vi "niRFUtil FWK Check Floating Point Range.vi"(0 "Upper Limit":dbl format="%#_6p", 1 "Upper Limit epsilon":dbl=1e-08, 2 "Lower Limit epsilon":dbl=1e-08, 5 "Lower Limit":dbl format="%#_6p", 7 "Value":dbl format="%#_6p", 11 "error in (no error)":errorcluster) -> (4 "In Range?":bool, 15 "error out":errorcluster)   [LabVIEW 2015, in "niRFUtil.lvlib"]
doc: "The default epsilon of 1E-7 works well for a range of numbers commonly seen in practice. However, for very large numbers and for small numbers a better epsilon should be chosen. Generally, if a number is greater than 0.1 and smaller than 1E+7, the default epsilon is probably fine.\n\nMachine epsilon for 64-bit floating point numbers (doubles) is between 1E-16 and 1E-17."
uses:
  niRFUtil.lvlib
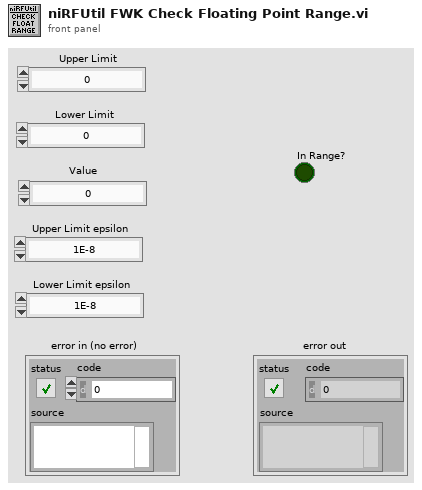
[diagram p1: front panel]
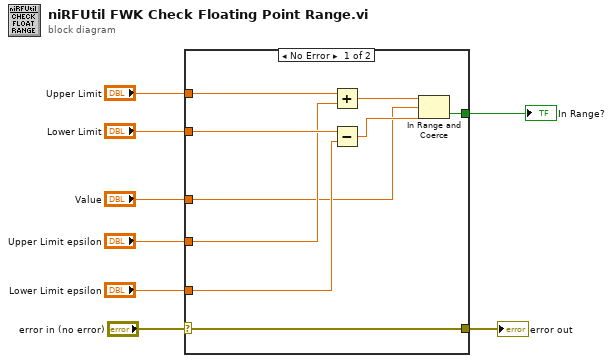
[diagram p0: block diagram]
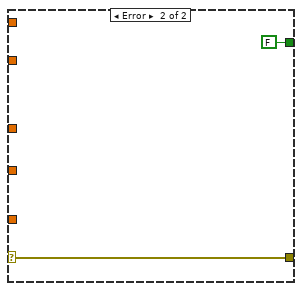
[diagram p2: hidden frame]
diagram:
  n1 = case shown="No Error" "error in (no error)" {
    selector: "error in (no error)" -> [w9 w18]
    tunnel: "Upper Limit" -> [w17 _]
    tunnel: "Lower Limit" -> [w16 _]
    tunnel: "Upper Limit epsilon" -> [w15 _]
    tunnel: "Lower Limit epsilon" -> [w14 _]
    tunnel: [w11 FALSE] -> w4
    tunnel: "Value" -> [w10 _]
    tunnel: [w9 w18] -> w1
    frame No Error {
      n2 = Add(x=w17, y=w15) -> (x+y=w13:dbl)
      n3 = Subtract(x=w16, y=w14) -> (x-y=w12:dbl)
      n4 = In Range and Coerce(upper limit=w13, x=w10, lower limit=w12) -> (In Range?=w11:bool)  [unwired: 1 out]
    }
    frame Error {
    }
  }
  "In Range?" <- w4
  "error out" <- w1
